vi "Top Level Controls.vi"() -> ()   [LabVIEW 2018]
uses:
  Program Files (x86)/National Instruments/LabVIEW 2018/examples/Design Patterns/State Machine/support/State Machine Fundamentals - State Enum.ctl
panel:
  in  "Close All Valves":bool
  in  "Fill Tank C":bool
  in  "Fill Tank B":bool
  in  "Stop":bool
  in  "Fill Tank A":bool
  in  "Vent Cycle":bool
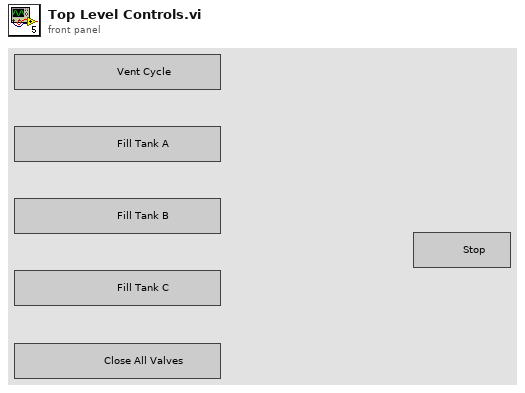
[diagram p1: front panel]
types:
  T1 = typedef "State Machine Fundamentals - State Enum.ctl" = enum16{"Initialize", "Wait for Event", "Vent Cycle", "Fill Tank A", "Fill Tank B", "Fill Tank C", "Close All Valves", "Stop"}
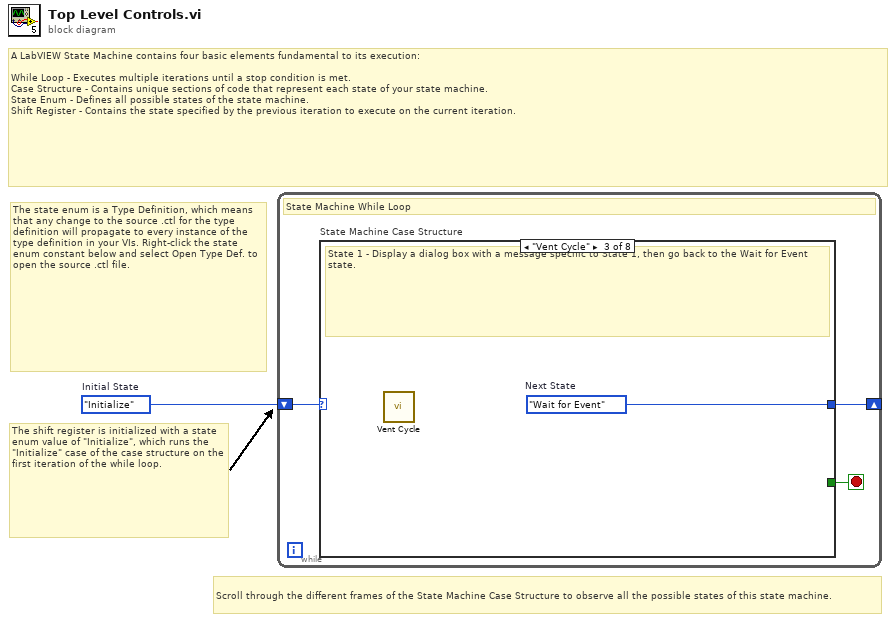
[diagram p0: block diagram]
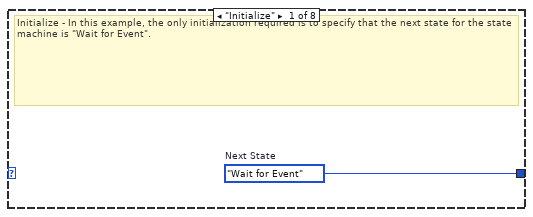
[diagram p2: hidden frame]
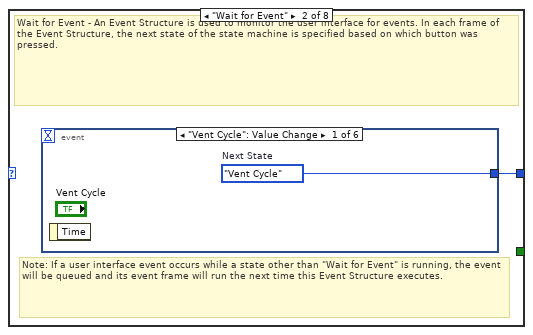
[diagram p3: hidden frame]
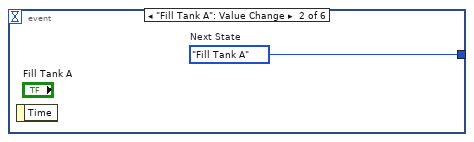
[diagram p4: hidden frame]
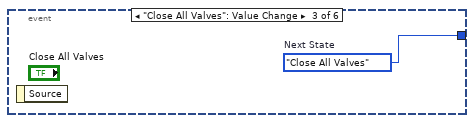
[diagram p5: hidden frame]
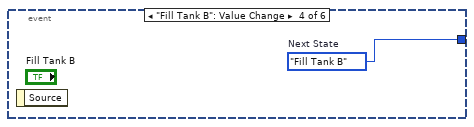
[diagram p6: hidden frame]
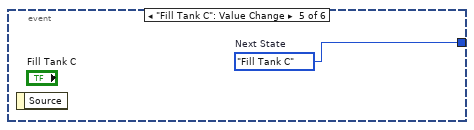
[diagram p7: hidden frame]
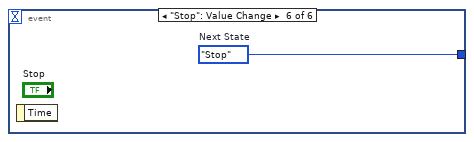
[diagram p8: hidden frame]
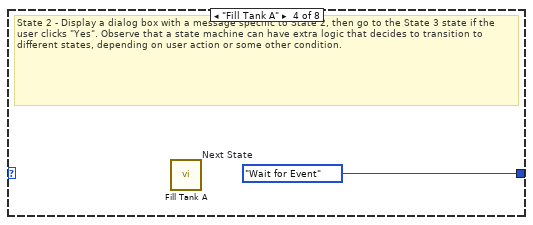
[diagram p9: hidden frame]
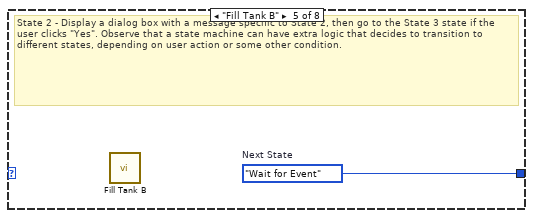
[diagram p10: hidden frame]
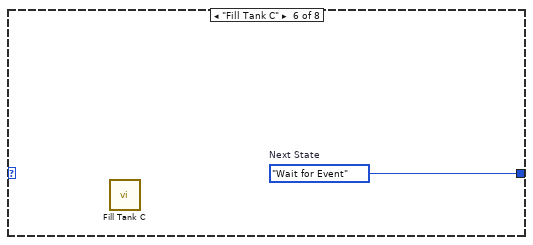
[diagram p11: hidden frame]
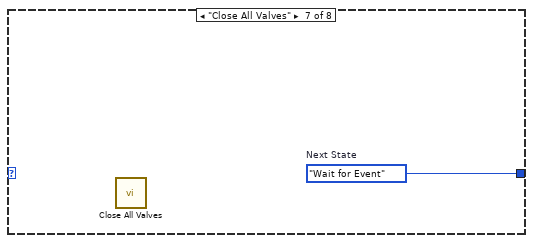
[diagram p12: hidden frame]
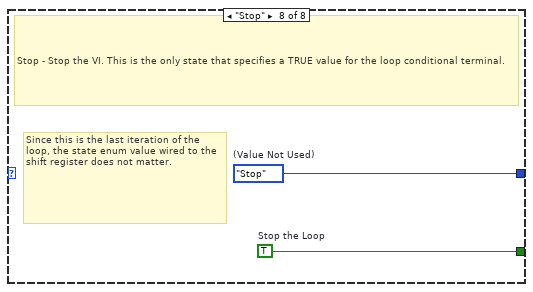
[diagram p13: hidden frame]
diagram:
  w1 = State_Machine_Fundamentals_-_State_Enum."Initialize"  # Initial State
  # "Scroll through the different frames of the State Machine Case Structure to observe all the possible states of this state machine."
  # "The state enum is a Type Definition, which means that any change to the source .ctl for the type definition will propagate to every instance of the type definition in your VIs. Right-click the state enum constant below and select Open Type Def. to open the source .ctl file."
  # "The shift register is initialized with a state enum value of \"Initialize\", which runs the \"Initialize\" case of the case structure on the first iteration of the while loop."
  # "A LabVIEW State Machine contains four basic elements fundamental to its execution:\n\nWhile Loop - Executes multiple iterations until a stop condition is met.\nCase Structure - Contains unique sections of code that represent each state of your state machine.\nState Enum - Defines all possible states of the state machine.\nShift Register - Contains the state specified by the previous iteration to execute on the current iteration."
  n1 = while {
    shift-right: [w3] -> _
    shift-left: w1 -> [w4]
    stop <- w2 stop-if-true
    # "State Machine While Loop"
    n2 = case "State Machine Case Structure" shown="\"Vent Cycle\"" w4 {
      tunnel: [w5 w6 w13 w14 w15 w16 w17 w19] -> w3
      tunnel: [_ _ _ _ _ _ _ w18] -> w2
      frame "Initialize" {
        w5 = State_Machine_Fundamentals_-_State_Enum."Wait for Event"  # Next State
        # "Initialize - In this example, the only initialization required is to specify that the next state for the state machine is \"Wait for Event\"."
      }
      frame "Wait for Event" {
        # "Note: If a user interface event occurs while a state other than \"Wait for Event\" is running, the event will be queued and its event frame will run the next time this Event Structure executes."
        # "Wait for Event - An Event Structure is used to monitor the user interface for events. In each frame of the Event Structure, the next state of the state machine is specified based on which button was pressed."
        n3 = event shown="[0] \"Vent Cycle\": Value Change" {
          selector: _ -> [_ _ _ _ _ _]
          dyn-events: _ -> [_ _ _ _ _ _]
          timeout: _ -> [_ _ _ _ _ _]
          tunnel: [w7 w8 w9 w10 w11 w12] -> w6
          event "Vent Cycle": Value Change {
            w7 = State_Machine_Fundamentals_-_State_Enum."Vent Cycle"  # Next State
            n4 = event-data() -> ()  [unwired: 1 in, 1 out]
          }
          event "Fill Tank A": Value Change {
            w8 = State_Machine_Fundamentals_-_State_Enum."Fill Tank A"  # Next State
            n5 = event-data() -> ()  [unwired: 1 in, 1 out]
          }
          event "Close All Valves": Value Change {
            w9 = State_Machine_Fundamentals_-_State_Enum."Close All Valves"  # Next State
            n6 = event-data() -> ()  [unwired: 1 in, 1 out]
          }
          event "Fill Tank B": Value Change {
            w10 = State_Machine_Fundamentals_-_State_Enum."Fill Tank B"  # Next State
            n7 = event-data() -> ()  [unwired: 1 in, 1 out]
          }
          event "Fill Tank C": Value Change {
            w11 = State_Machine_Fundamentals_-_State_Enum."Fill Tank C"  # Next State
            n8 = event-data() -> ()  [unwired: 1 in, 1 out]
          }
          event "Stop": Value Change {
            w12 = State_Machine_Fundamentals_-_State_Enum."Stop"  # Next State
            n9 = event-data() -> ()  [unwired: 1 in, 1 out]
          }
        }
      }
      frame "Vent Cycle" {
        w13 = State_Machine_Fundamentals_-_State_Enum."Wait for Event"  # Next State
        # "State 1 - Display a dialog box with a message specific to State 1, then go back to the Wait for Event state."
        n10 = call "Vent Cycle.vi"() -> ()  [unwired: 12 in]
      }
      frame "Fill Tank A" {
        w14 = State_Machine_Fundamentals_-_State_Enum."Wait for Event"  # Next State
        # "State 2 - Display a dialog box with a message specific to State 2, then go to the State 3 state if the user clicks \"Yes\". Observe that a state machine can have extra logic that decides to transition to different states, depending on user action or some other condition."
        n11 = call "Fill Tank A.vi"() -> ()  [unwired: 12 in]
      }
      frame "Fill Tank B" {
        w15 = State_Machine_Fundamentals_-_State_Enum."Wait for Event"  # Next State
        # "State 2 - Display a dialog box with a message specific to State 2, then go to the State 3 state if the user clicks \"Yes\". Observe that a state machine can have extra logic that decides to transition to different states, depending on user action or some other condition."
        n12 = call "Fill Tank B.vi"() -> ()  [unwired: 12 in]
      }
      frame "Fill Tank C" {
        w16 = State_Machine_Fundamentals_-_State_Enum."Wait for Event"  # Next State
        n13 = call "Fill Tank C.vi"() -> ()  [unwired: 12 in]
      }
      frame "Close All Valves" {
        w17 = State_Machine_Fundamentals_-_State_Enum."Wait for Event"  # Next State
        n14 = call "Close All Valves.vi"() -> ()  [unwired: 12 in]
      }
      frame "Stop" {
        w18 = TRUE  # Stop the Loop
        w19 = State_Machine_Fundamentals_-_State_Enum."Stop"  # (Value Not Used)
        # "Since this is the last iteration of the loop, the state enum value wired to the shift register does not matter."
        # "Stop - Stop the VI. This is the only state that specifies a TRUE value for the loop conditional terminal."
      }
    }
  }
